vi "PQprotocolVersion.vi"(8 "error in (no error)":errorcluster, 10 "conn":u32) -> (0 "error out":errorcluster, 3 "PQprotocolVersion":u32)   [LabVIEW 2017, in "libpqlv.lvlib"]
doc: "Interrogates the frontend/backend protocol being used."
uses:
  libpqlv.lvlib
  lib/libpq.dll
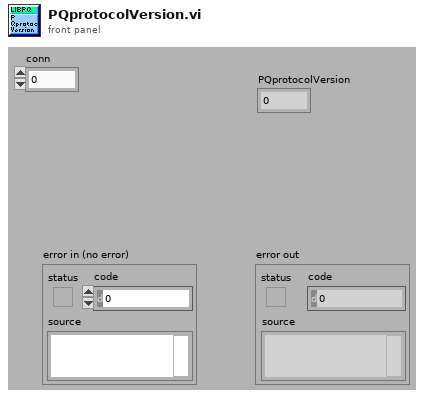
[diagram p1: front panel]
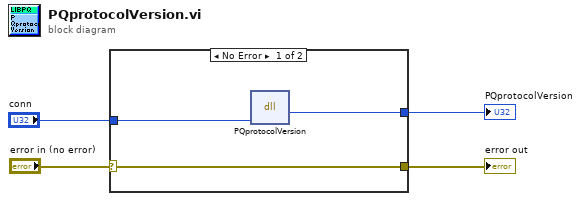
[diagram p0: block diagram]
diagram:
  n1 = case shown="No Error" "error in (no error)" {
    selector: "error in (no error)" -> [w7 w8]
    tunnel: [w7 w8] -> w3
    tunnel: [w6 _] -> w2
    tunnel: "conn" -> [w5 _]
    frame No Error {
      n2 = dll-call lib="D:/Users/erics/Documents/active/DAQ/PostgreSQL2LabVIEW/libpqlv/lib/libpq.*" fn="PQprotocolVersion"("conn"=w5) -> ("PQprotocolVersion"=w6:u32)  [unwired: 4 in, 2 out]
    }
    frame Error {
    }
  }
  "PQprotocolVersion" <- w2
  "error out" <- w3
